vi "Home.SetSubpanelRef.vi"(8 "error in (no error)":errorcluster, 10 "Subpanel Ref":refnum<vi>, 11 "Home":refnum<class "Home.lvclass">) -> (0 "error out":errorcluster, 3 "Home out":refnum<class "Home.lvclass">)   [LabVIEW 2022 SP3, in "Home.lvclass"]
uses:
  Home.lvclass
  Home.lvclass/Home.ctl
panel:
  # "For instructions on how to use the JKI State Machine Objects, examples and video tutorials, visit:\nhttp://jki.net/state-machine-objects/\n\nJKI State Machine Objects™\nhttp://jki.net/state-machine-objects/\nCopyright (C) 2005-2015, JKI <info@jki.net>\nALL RIGHTS RESERVED"
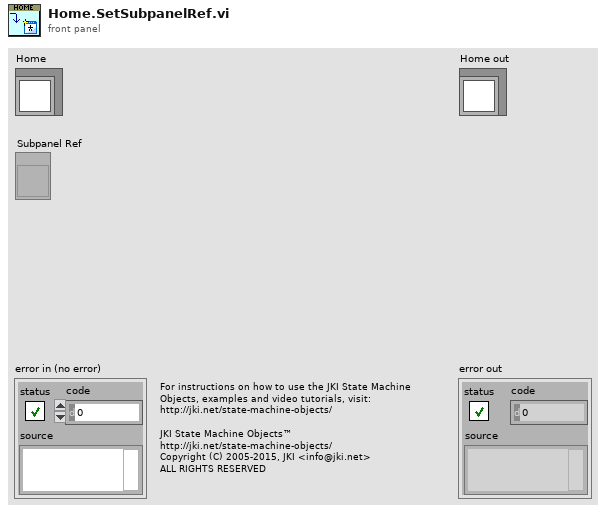
[diagram p1: front panel]
types:
  T1 = typedef "Home.lvclass/PrivateData--Ref.ctl" = refnum<data-value>
  T2 = typedef "Home.lvclass/PrivateData--Cluster.ctl" = cluster{"Public Events":T3, "Subpanel Ref":refnum<vi>, "UI State":T4}
  T3 = typedef "Home.lvclass/PublicEvents--Cluster.ctl" = cluster{"UI State":refnum<user-event>}
  T4 = typedef "Home.lvclass/SMO.UI_Embed State--enum.ctl" = enum16{"unknown", "Opened", "Embedded", "Closed"}
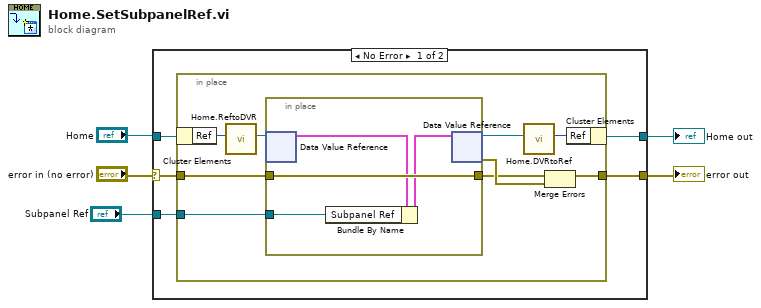
[diagram p0: block diagram]
diagram:
  n1 = case shown="No Error" "error in (no error)" {
    selector: "error in (no error)" -> [w9 w25]
    tunnel: [w8 w25] -> w2
    tunnel: [w7 w24] -> w4
    tunnel: "Home" -> [w10 w24]
    tunnel: "Subpanel Ref" -> [w6 _]
    frame No Error {
      n2 = in-place {
        in-place-border: w9 -> [w19]
        in-place-border: [w16] -> w8
        in-place-border: w6 -> [w11]
        n3 = in-place-cluster #1(w10) -> ("Ref"=w13:u32)
        n4 = call "Home.ReftoDVR.vi"("Ref"=w13) -> ("Ref"=w12:T1)  [unwired: 10 in]
        n5 = in-place {
          in-place-border: w19 -> [w23]
          in-place-border: [w23] -> w17
          in-place-border: w11 -> [w20]
          n6 = in-place-dvr #2(w12) -> (w22:T2)  [unwired: 1 out]
          n7 = Bundle By Name(cluster=w22, "Subpanel Ref"=w20) -> (w21:T2)
          n8 = in-place-dvr #2(w21) -> (w15:T1, w18:errorcluster)
        }
        n9 = call "Home.DVRtoRef.vi"("Ref"=w15) -> ("Ref"=w14:u32)  [unwired: 10 in]
        n10 = Merge Errors(w17, w18) -> (w16:errorcluster)
        n11 = in-place-cluster #1("Ref"=w14) -> (w7:refnum<class "Home.lvclass">)
      }
    }
    frame Error {
    }
  }
  "error out" <- w2
  "Home out" <- w4
